vi "Utility Read Binary Block Data.vi"(6 "Error In":errorcluster, 9 "VISA In":refnum<visa-resource-name>) -> (0 "Error Out":errorcluster, 2 "Data":string, 3 "VISA Out":refnum<visa-resource-name>)   [LabVIEW 2015]
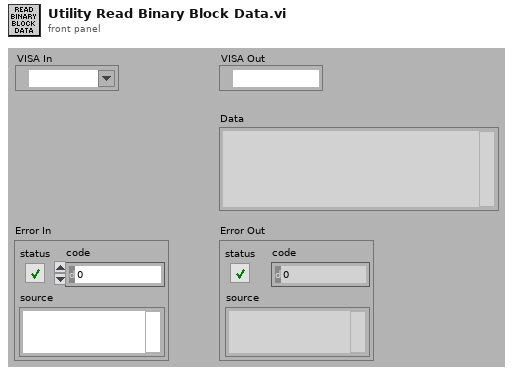
[diagram p1: front panel]
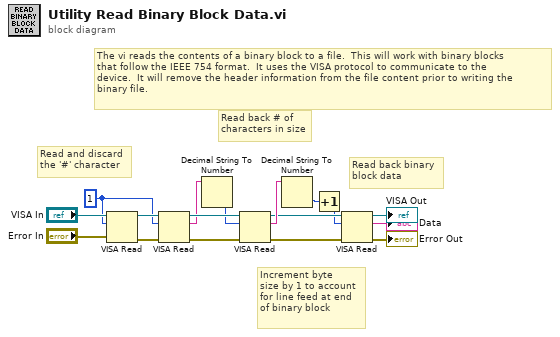
[diagram p0: block diagram]
diagram:
  w3 = u32 1 ("byte count")
  # "The vi reads the contents of a binary block to a file.  This will work with binary blocks\nthat follow the IEEE 754 format.  It uses the VISA protocol to communicate to the\ndevice.  It will remove the header information from the file content prior to writing the\nbinary file."
  # "Read back binary\nblock data"
  # "Increment byte\nsize by 1 to account\nfor line feed at end\nof binary block"
  # "Read back # of\ncharacters in size"
  # "Read and discard\nthe '#' character"
  n1 = VISA Read(VISA resource name="VISA In", byte count=w3, error in (no error)="Error In") -> (VISA resource name out=w9:refnum<visa-resource-name>, error out=w6:errorcluster)  [unwired: 2 out]
  n2 = VISA Read(VISA resource name=w9, byte count=w3, error in (no error)=w6) -> (VISA resource name out=w11:refnum<visa-resource-name>, read buffer=w10:string, error out=w12:errorcluster)  [unwired: 1 out]
  n3 = Decimal String To Number(string=w10) -> (number=w2:i32)  [unwired: 2 in, 1 out]
  n4 = VISA Read(VISA resource name=w11, byte count=w2, error in (no error)=w12) -> (VISA resource name out=w13:refnum<visa-resource-name>, read buffer=w14:string, error out=w7:errorcluster)  [unwired: 1 out]
  n5 = Decimal String To Number(string=w14) -> (number=w15:i32)  [unwired: 2 in, 1 out]
  n6 = Increment(x=w15) -> (x+1=w1:i32)
  n7 = VISA Read(VISA resource name=w13, byte count=w1, error in (no error)=w7) -> (VISA resource name out=→"VISA Out":refnum<visa-resource-name>, read buffer=→"Data":string, error out=→"Error Out":errorcluster)  [unwired: 1 out]
